vi "use photons for state.vi"(0 "state in":T1, 1 "apply measurement?":bool, 5 "location":T3, 7 "z-offset":i16, 9 "half valid z-range (ncycles * 64)":i16=500) -> (4 "use photons to update tracker?":bool, 8 "on target":bool)   [LabVIEW 2010]
uses:
  kalman 3-axis state.ctl
  integrating single axis kalman state.ctl
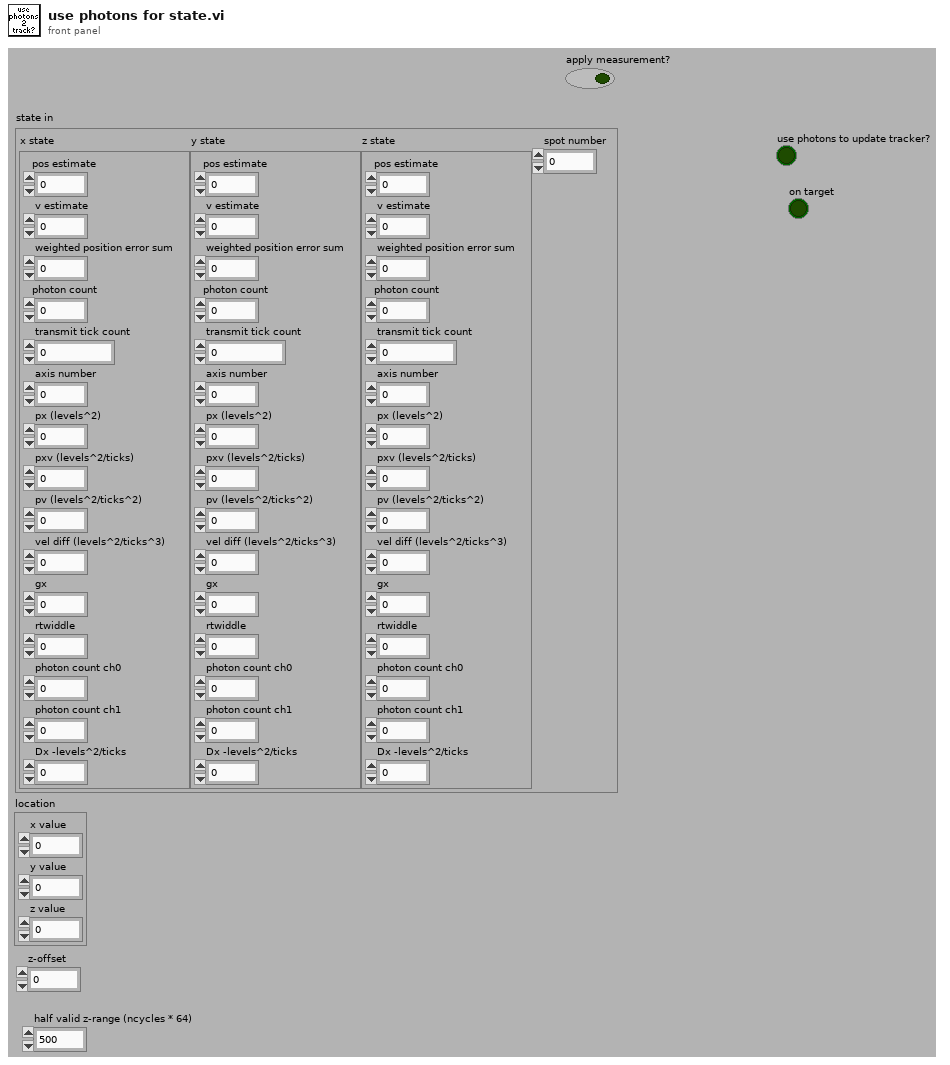
[diagram p1: front panel]
types:
  T1 = typedef "kalman 3-axis state.ctl" = cluster{"x state":T2, "y state":T2, "z state":T2, "spot number":u8}
  T2 = typedef "integrating single axis kalman state.ctl" = cluster{"pos estimate":fxp<+/-,32,16>, "v estimate":fxp<+/-,16,0>, "weighted position error sum":fxp<+/-,32,32>, "photon count":u32, "transmit tick count":u32, "axis number":u8, "px (levels^2)":fxp<+,32,19>, "pxv (levels^2/ticks)":fxp<+,32,2>, "pv (levels^2/ticks^2)":fxp<+,32,-14>, "vel diff (levels^2/ticks^3)":fxp<+,24,-22>, "gx":fxp<+,16,8>, "rtwiddle":fxp<+,16,26>, "photon count ch0":u32, "photon count ch1":u32, "Dx -levels^2/ticks":fxp<+,32,19>}
  T3 = cluster{"x value":i16, "y value":i16, "z value":i16}
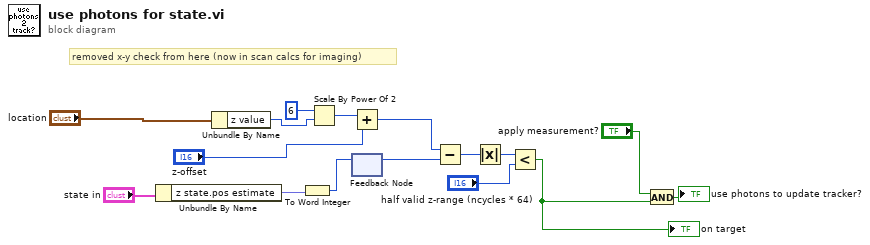
[diagram p0: block diagram]
diagram:
  # "removed x-y check from here (now in scan calcs for imaging)"
  n1 = Unbundle By Name("state in") -> ("z state.pos estimate"=w6:fxp<+/-,32,16>)
  n2 = Unbundle By Name("location") -> ("z value"=w9:i16)
  n3 = To Word Integer(number=w6) -> (16bit integer=w14:i16)
  n4 = Scale By Power Of 2(n=6, x=w9) -> (x*2^n=w8:i16)
  n5 = Add(x=w8, y="z-offset") -> (x+y=w7:i16)
  n6 = feedback-in #1(w14) -> ()
  n7 = feedback #1() -> (w2:i16)  [unwired: 1 in]
  n8 = Subtract(x=w7, y=w2) -> (x-y=w13:i16)
  n9 = Absolute Value(x=w13) -> (abs(x)=w12:i16)
  n10 = Less?(x=w12, y="half valid z-range (ncycles * 64)") -> (x < y?=w4:bool)
  "on target" <- w4
  n11 = And(x="apply measurement?", y=w4) -> (x .and. y?=→"use photons to update tracker?":bool)
